vi "ziExample-PollData.vi"(0 "Address":string="DEV", 1 "stop":bool, 5 "Save":bool) -> (17 "theta (deg)":dbl[](array[numeric]), 20 "Selected Device":string, 21 "Demod R (V)":dbl format="%_4p", 22 "Demod Phi (deg)":dbl format="%.3p", 23 "Spectral Density\nVrms/sqrt(Hz)":dbl=1.331104953906021e-08 format="%0.2p", 24 "Savedas":string, 25 "Demod Sample Out":T3 {"Aux In 1 (V)" format="%#_5p"; "Aux In 0 (V)" format="%#_5p"; "X (Vrms)" format="%#_5p"; "Y (Vrms)" format="%#_5p"; "Osc Phase (rad)" format="%#.3g"}, 26 "DIO Out":T2, 27 "AuxIn Out":T1)   [LabVIEW 2009]
doc: "Control a Zurich instrument device via the LabOne Labview API. \nRequirements: Zurich Instruments MFLI, HF2 or UHFLI \nThis example polls data from the instrument.\n\n© Zurich Instruments AG, www.zhinst.com"
uses:
  <instrlib>/Zurich Instruments LabOne/Public/Data/ziTypePollType.ctl
  <instrlib>/Zurich Instruments LabOne/Public/Data/ziTypeDemodSampleEx.ctl
  <instrlib>/Zurich Instruments LabOne/Public/Data/ziTypeAuxInSample.ctl
  <instrlib>/Zurich Instruments LabOne/Public/Configure/ziSetValueDoubleArray.vi
  <instrlib>/Zurich Instruments LabOne/Public/Data/ziGetEventAuxInSample.vi
  <instrlib>/Zurich Instruments LabOne/Public/Data/ziGetEventDemodSample.vi
  <instrlib>/Zurich Instruments LabOne/Public/Data/ziGetEventDIOSample.vi
  <instrlib>/Zurich Instruments LabOne/Zurich Instruments LabOne.lvlib
panel:
  out "data":cluster{dbl[], u32[], dbl[]}
  out "Error Out":errorcluster
  in  "Saveas":path
  in  "Edge":u16(ring)=1 items=["Off", "Rising Edge", "Falling Edge", "Both Edges"]
  in  "DIO Channel":u16(ring) items=["Continous"=0, "DIO 0 / Tigger 3"=1, "DIO 1 / Tigger 4"=4, "DIO 0|1 / Tigger 3|4"=5]
  in  "binSave":bool caption="Binary Save"
  out "Buffer Overflow":bool
  out "Demod sample":dbl[](graph)
  out "ziValueType":T4
  out "DIO":u32[](graph)
  out "AUX Input":dbl[](graph)
  # "ziExample-PollData.vi\nRequirements: HF2, UHFLI or MFLI\nsee block diagram for VI description"
  # "Tested Instruments:\n- MFLI\n- HF2LI\n- UHFLI"
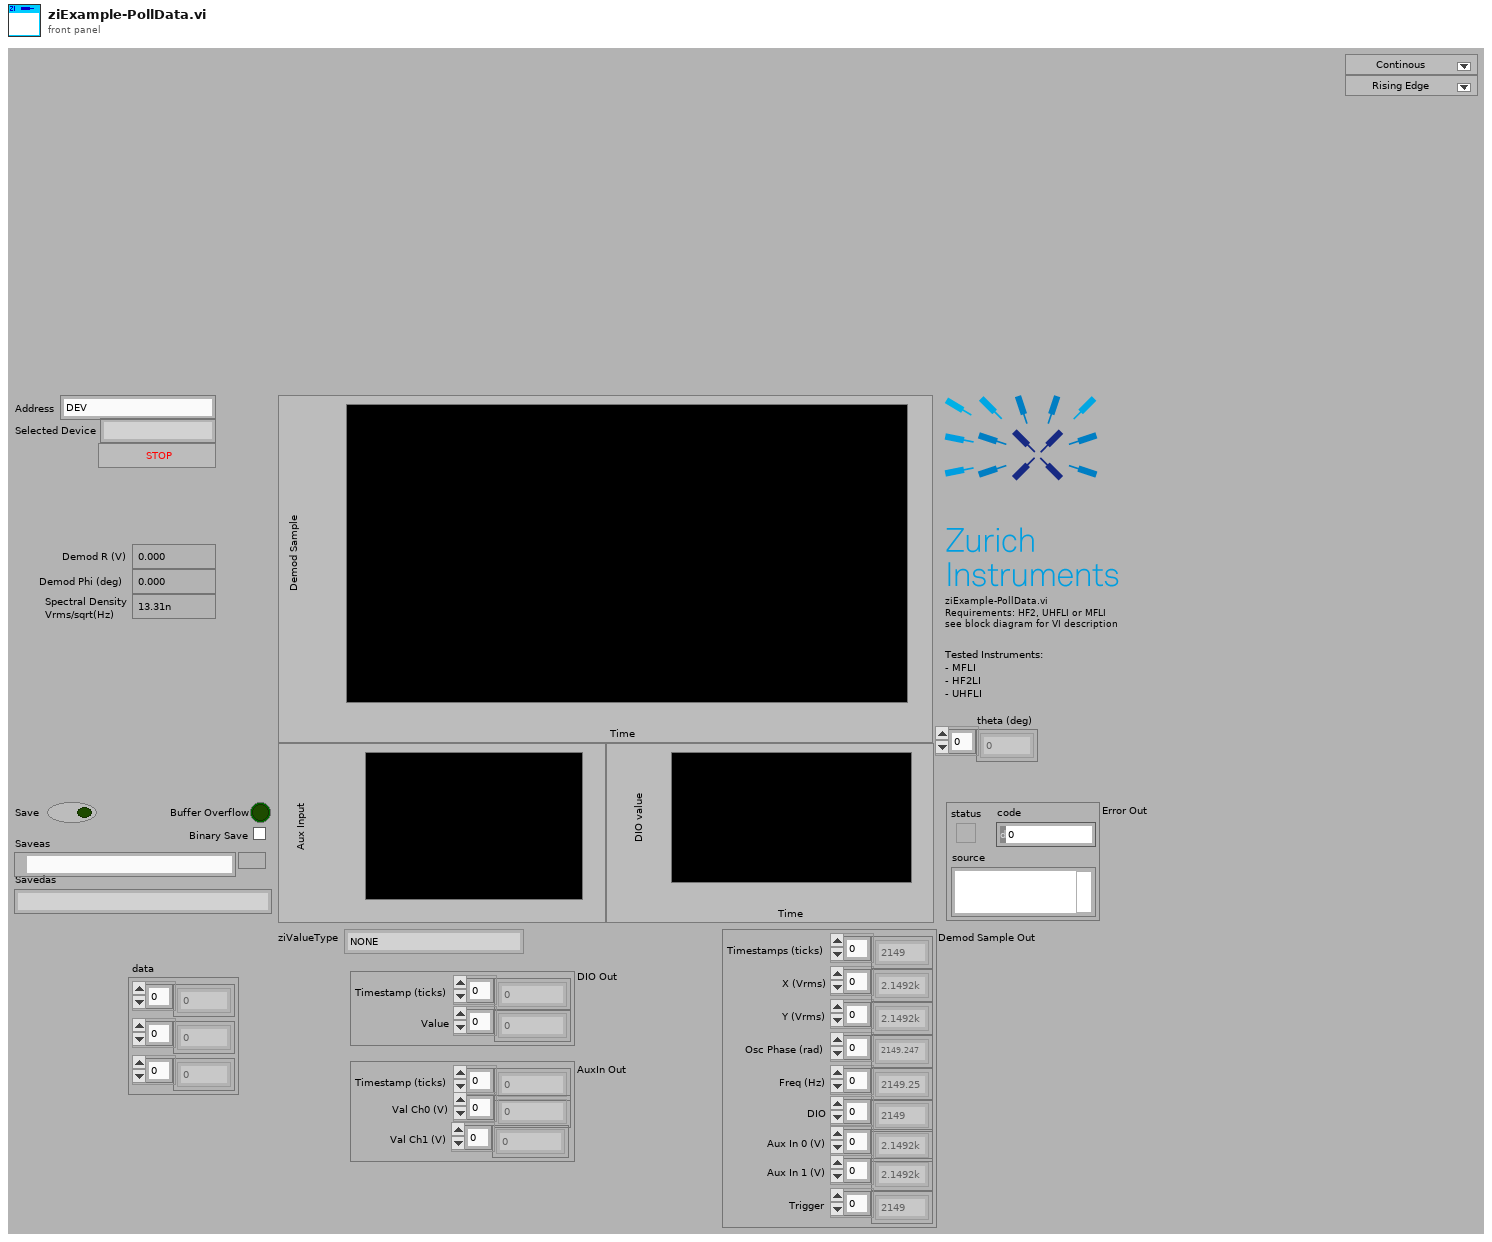
[diagram p1: front panel]
types:
  T1 = typedef "Zurich Instruments LabOne.lvlib/ziTypeAuxInSample.ctl" = cluster{"Timestamp (ticks)":u64[], "Val Ch0 (V)":dbl[], "Val Ch1 (V)":dbl[]}
  T2 = cluster{"Timestamp (ticks)":u64[], "Value":u32[]}
  T3 = typedef "ziTypeDemodSampleEx.ctl" = cluster{"Timestamps (ticks)":u64[], "X (Vrms)":dbl[], "Y (Vrms)":dbl[], "Osc Phase (rad)":dbl[], "Freq (Hz)":dbl[], "DIO":u32[], "Aux In 0 (V)":dbl[], "Aux In 1 (V)":dbl[], "Trigger":u32[]}
  T4 = typedef "Zurich Instruments LabOne.lvlib/ziTypePollType.ctl" = enum16{"NONE", "DOUBLE_DATA", "INTEGER_DATA", "DEMOD_SAMPLE", "SCOPE_WAVE_HF2", "AUXIN_SAMPLE", "DIO_SAMPLE", "BYTE_ARRAY", "PWA_WAVE", "9", "10", "11", "12", "13", "14", "15", "TREE_CHANGE_DEPRI", "17", "ERROR", "19", "20", "21", "22", "23", "24", "25", "26", "27", "28", "29", "30", "31", "DOUBLE_DATA_TS", "INTEGER_DATA_TS", "34", "SCOPE_WAVE", "36", "37", "BYTE_ARRAY_TS", "39", "40", "41", "42", "43", "44", "45", "CNT_DATA", "47", "TREE_CHANGE", "49", "50", "51", "52", "53", "54", "55", "56", "57", "58", "59", "60", "61", "62", "63", "SWEEPER_DATA", "SPECTRUM_DATA", "ADVISOR_DATA", "67", "IMP_DATA"}
  T5 = typedef "Zurich Instruments LabOne.lvlib/ziTypeHandle.ctl" = cluster{"handleValid":bool, "Conn":u64, "Path Prefix":string, "Handle":u64, "Connected":bool, "Clockbase(s)":dbl}
  T6 = enum16{"open", "replace", "create", "open or create", "replace or create", "replace or create with confirmation"}
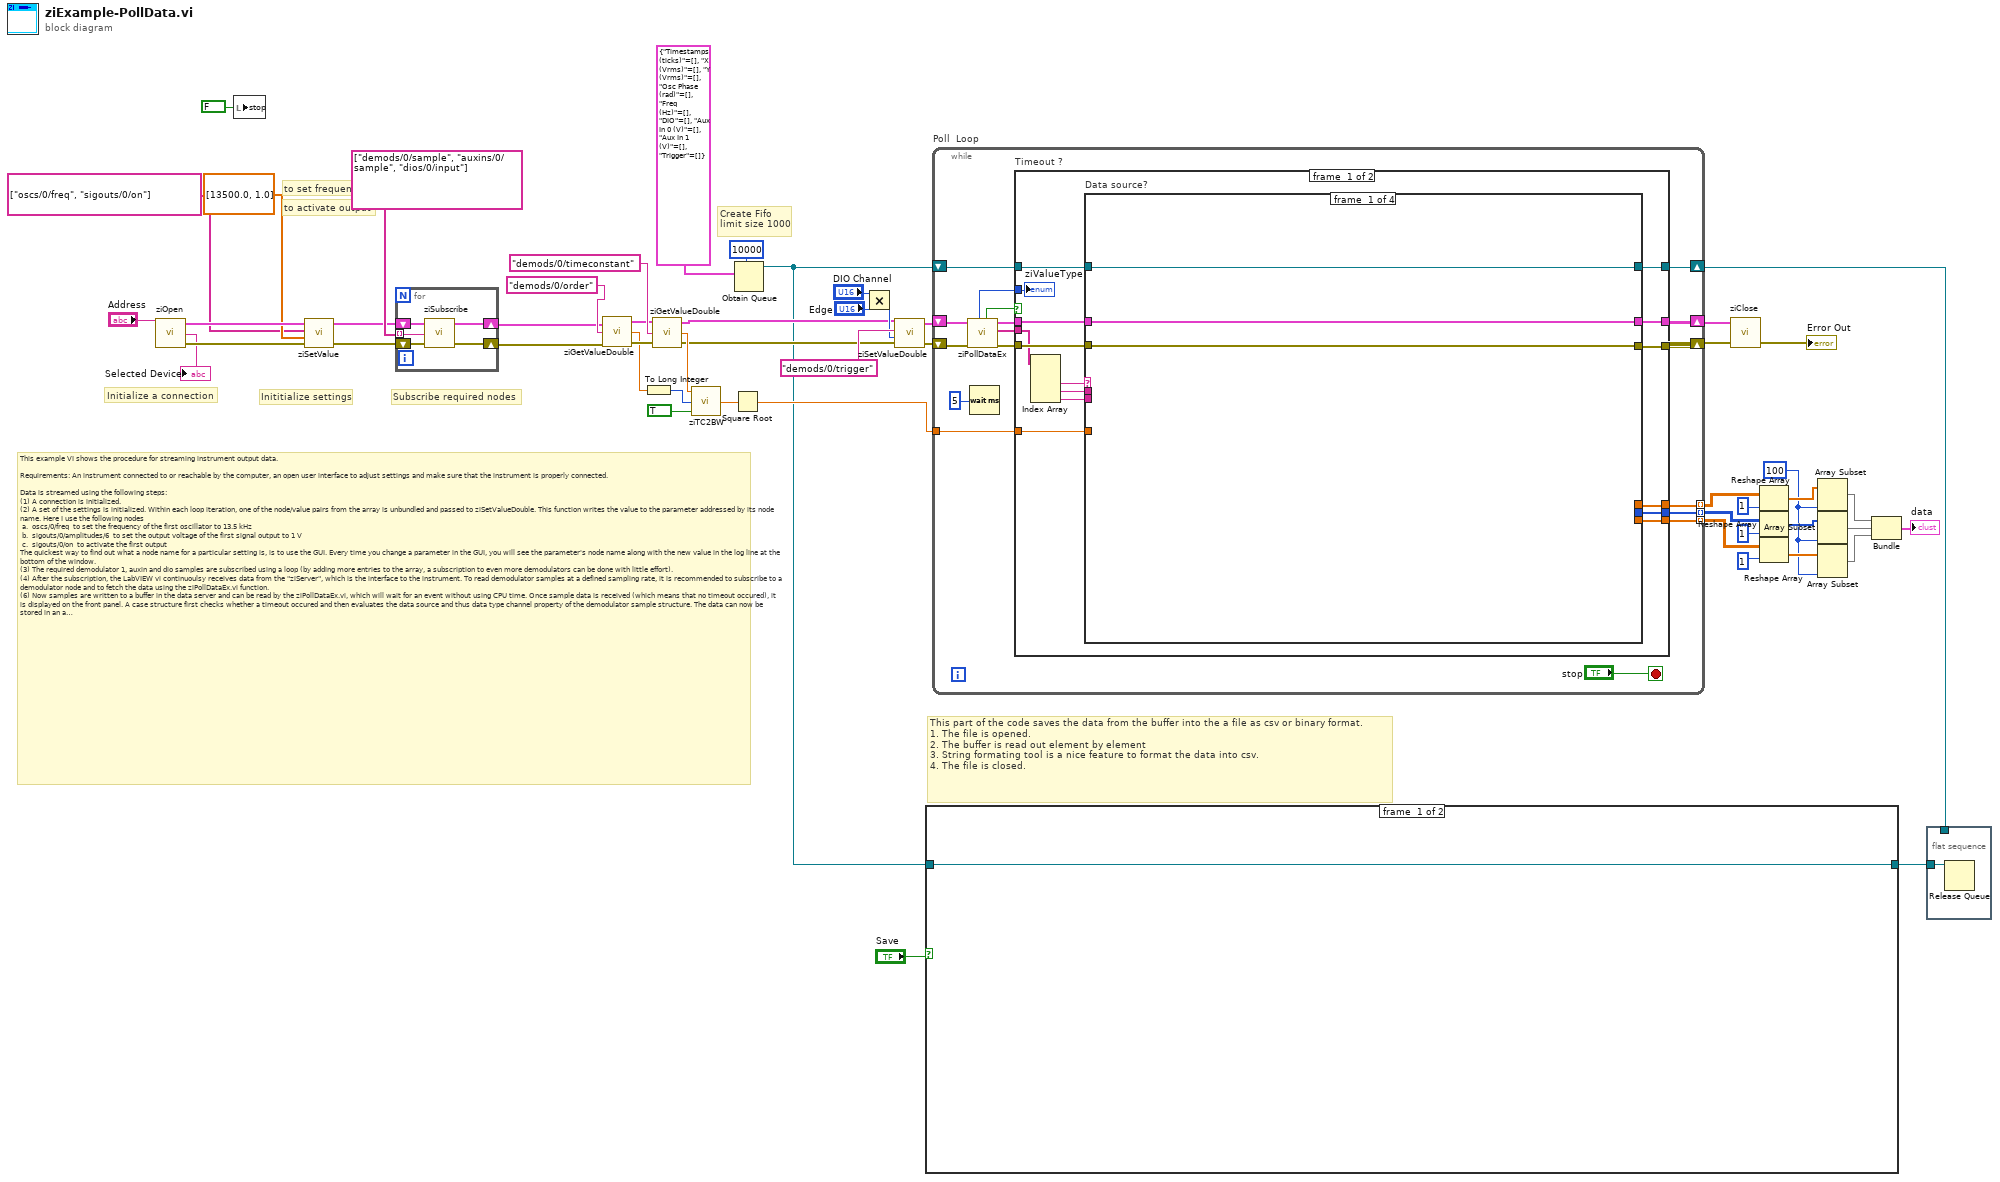
[diagram p0: block diagram]
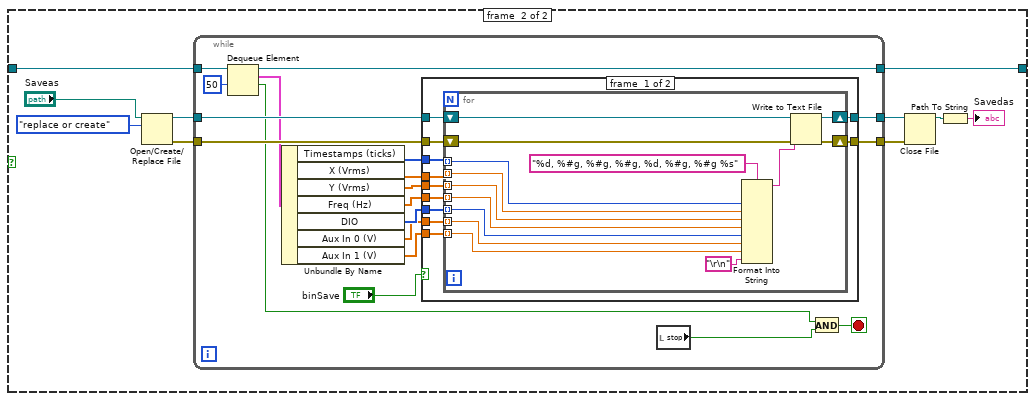
[diagram p2: hidden frame]
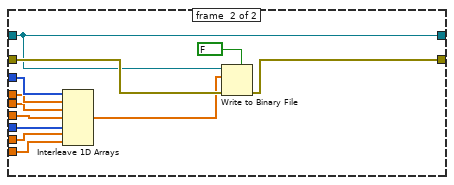
[diagram p3: hidden frame]
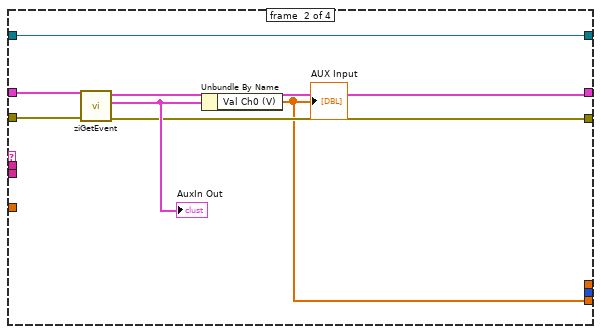
[diagram p4: hidden frame]
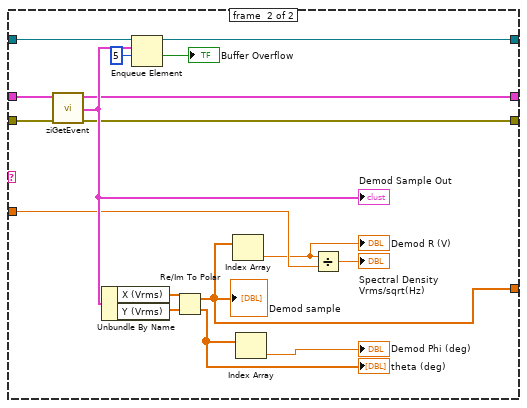
[diagram p7: hidden frame]
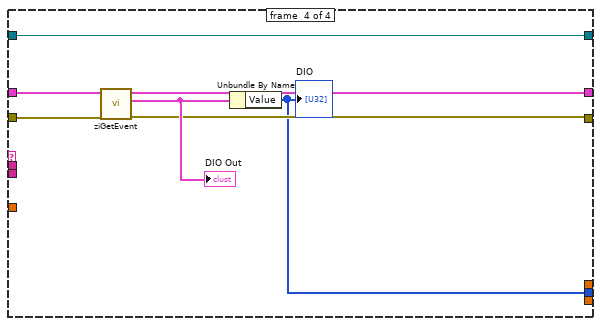
[diagram p8: hidden frame]
diagram:
  w2 = 100 ("dimension size")
  # "This part of the code saves the data from the buffer into the a file as csv or binary format. \n1. The file is opened.\n2. The buffer is read out element by element\n3. String formating tool is a nice feature to format the data into csv.\n4. The file is closed."
  # "Create Fifo\nlimit size 1000"
  # "to activate output"
  # "to set frequency"
  # "Inititialize settings"
  # "Initialize a connection"
  # "Subscribe required nodes"
  # "This example VI shows the procedure for streaming instrument output data.\n\nRequirements: An instrument connected to or reachable by the computer, an open user interface to adjust settings and make sure that the instrument is properly connected. \n\nData is streamed using the following steps:\n(1) A connection is initialized.\n(2) A set of the settings is initialized. Within each loop iteration, one of the node/value pairs from the array is unbundled and passed to ziSetValueDouble. This function writes the value to the parameter addressed by its node name. Here I use the following nodes\n a. \toscs/0/freq \tto set the frequency of the first oscillator to 13.5 kHz\n b. \tsigouts/0/amplitudes/6 \tto set the output voltage of the first signal output to 1 V\n c. \tsigouts/0/on \tto activate the first output\nThe quickest way to find out what a node name for a particular setting is, is to use the GUI. Every time you change a parameter in the GUI, you will see the parameter's node name along with the new value in the log line at the bottom of the window. \n(3) The required demodulator 1, auxin and dio samples are subscribed using a loop (by adding more entries to the array, a subscription to even more demodulators can be done with little effort).\n(4) After the subscription, the LabVIEW vi continuoulsy receives data from the \"ziServer\", which is the interface to the instrument. To read demodulator samples at a defined sampling rate, it is recommended to subscribe to a demodulator node and to fetch the data using the ziPollDataEx.vi function. \n(6) Now samples are written to a buffer in the data server and can be read by the ziPollDataEx.vi, which will wait for an event without using CPU time. Once sample data is received (which means that no timeout occured), it is displayed on the front panel. A case structure first checks whether a timeout occured and then evaluates the data source and thus data type channel property of the demodulator sample structure. The data can now be stored in an array or a queue or be shown in a waveform chart. \n(7) Finally, the connection is closed. \n \n© Zurich Instruments AG, 2016, www.zhinst.com"
  n1 = call <instrlib>:"ziOpen.vi"("Address"="Address") -> ("Error Out"=w49:errorcluster, "Selected Device"=→"Selected Device":string, "HandleOut"=w48:T5)  [unwired: 1 in, 2 out]
  n2 = local write "stop"(FALSE ("stop")) -> ()
  n3 = call-poly <instrlib>:"ziSetValue.vi"("Error In"=w49, "Values"=dbl[] [13500.0, 1.0], "Paths"=string[] ["oscs/0/freq", "sigouts/0/on"], "Handle In"=w48) -> ("Error Out"=w50:errorcluster, "Handle Out"=w51:T5)  [unwired: 1 in]
  n4 = for {
    shift-right: [w58] -> w32
    shift-left: w51 -> [w56]
    shift-right: [w57] -> w31
    shift-left: w50 -> [w55]
    tunnel: string[] ["demods/0/sample", "auxins/0/sample", "dios/0/input"] -> [w54] mode=indexing
    n5 = call <instrlib>:"ziSubscribe.vi"("error in"=w55, "Path ()"=w54, "Handle In"=w56) -> ("error out"=w57:errorcluster, "Handle Out"=w58:T5)  [unwired: 1 in]
  }
  n6 = call <instrlib>:"ziGetValueDouble.vi"("error in"=w31, "Path"="demods/0/order", "Handle in"=w32) -> ("error out"=w38:errorcluster, "Value"=w37:dbl, "Handle out"=w39:T5)
  n7 = To Long Integer(number=w37) -> (32bit integer=w36:i32)
  n8 = call <instrlib>:"ziGetValueDouble.vi"("error in"=w38, "Path"="demods/0/timeconstant", "Handle in"=w39) -> ("error out"=w19:errorcluster, "Value"=w35:dbl, "Handle out"=w20:T5)
  n9 = call <instrlib>:"ziTC2BW.vi"("Eq BW (F)"=TRUE ("Eq BW"), "Order (1)"=w36, "TC (s)"=w35) -> ("BW (Hz)"=w34:dbl)
  n10 = Square Root(x=w34) -> (sqrt(x)=w30:dbl)
  n11 = Obtain Queue(max queue size (-1, unlimited)=10000, element data type=T3 {"Timestamps (ticks)"=[], "X (Vrms)"=[], "Y (Vrms)"=[], "Osc Phase (rad)"=[], "Freq (Hz)"=[], "DIO"=[], "Aux In 0 (V)"=[], "Aux In 1 (V)"=[], "Trigger"=[]} ("Demod Sample Out")) -> (queue out=w18:refnum<queue>)  [unwired: 3 in, 2 out]
  n12 = Multiply(x="DIO Channel", y="Edge") -> (x*y=w25:u16)
  n13 = call <instrlib>:"ziSetValueDouble.vi"("Error In"=w19, "Value"=w25, "Path"="demods/0/trigger", "Handle In"=w20) -> ("Error Out"=w22:errorcluster, "Handle Out"=w21:T5)  [unwired: 1 in]
  n14 = case shown="True" "Save" {
    tunnel: w18 -> [w59 w69]
    tunnel: [w59 w64] -> w28
    frame #0 {
    }
    frame #1 {
      n15 = Open/Create/Replace File(file path (use dialog)="Saveas", operation (0:open)=T6."replace or create") -> (refnum out=w67:refnum<file>, error out=w68:errorcluster)  [unwired: 4 in, 1 out]
      n16 = while {
        tunnel: w68 -> [w81]
        tunnel: w67 -> [w80]
        tunnel: [w79] -> w66
        tunnel: [w78] -> w65
        tunnel: [w73] -> w64
        tunnel: w69 -> [w75]
        stop <- w71 stop-if-true
        n17 = Dequeue Element(queue=w75, timeout in ms (-1)=50) -> (queue out=w73:refnum<queue>, element=w76:T3, timed out?=w74:bool)  [unwired: 1 in, 1 out]
        n18 = Unbundle By Name(w76) -> ("Timestamps (ticks)"=w88:u64[], "X (Vrms)"=w85:dbl[], "Y (Vrms)"=w87:dbl[], "Freq (Hz)"=w86:dbl[], "DIO"=w84:u32[], "Aux In 0 (V)"=w83:dbl[], "Aux In 1 (V)"=w82:dbl[])
        n19 = case shown="False" "binSave" {
          tunnel: w88 -> [w99 w121]
          tunnel: w87 -> [w98 w119]
          tunnel: w86 -> [w97 w118]
          tunnel: w85 -> [w96 w120]
          tunnel: w84 -> [w95 w117]
          tunnel: w83 -> [w94 w116]
          tunnel: w82 -> [w93 w115]
          tunnel: w81 -> [w92 w124]
          tunnel: w80 -> [w91 w122]
          tunnel: [w90 w123] -> w79
          tunnel: [w89 w122] -> w78
          frame #0 {
            n20 = for {
              tunnel: w99 -> [w107] mode=indexing
              tunnel: w98 -> [w105] mode=indexing
              tunnel: w96 -> [w106] mode=indexing
              shift-right: [w112] -> w89
              shift-left: w91 -> [w113]
              tunnel: w97 -> [w104] mode=indexing
              shift-right: [w111] -> w90
              shift-left: w92 -> [w110]
              tunnel: w95 -> [w102] mode=indexing
              tunnel: w94 -> [w101] mode=indexing
              tunnel: w93 -> [w103] mode=indexing
              n21 = Format Into String(format string="%d, %#g, %#g, %#g, %d, %#g, %#g %s", w107, w106, w105, w104, w102, w101, w103, "\r\n") -> (resulting string=w100:string)  [unwired: 2 in, 1 out]
              n22 = Write to Text File(file (use dialog)=w113, text=w100, error in=w110) -> (refnum out=w112:refnum<file>, error out=w111:errorcluster)  [unwired: 2 out]
            }
          }
          frame #1 {
            n23 = Interleave 1D Arrays(w121, w120, w119, w118, w117, w116, w115) -> (w114:dbl[])
            n24 = Write to Binary File(file (use dialog)=w122, data=w114, error in=w124, 5:FALSE ("prepend array or string size? (T)")) -> (error out=w123:errorcluster)  [unwired: 4 out]
          }
        }
        n25 = local read "stop"() -> (w72:bool)
        n26 = And(x=w74, y=w72) -> (x .and. y?=w71:bool)
      }
      n27 = Close File(refnum=w65, error in=w66) -> (path=w61:path)  [unwired: 1 out]
      n28 = Path To String(path=w61) -> (string=→"Savedas":string)
    }
  }
  n29 = while "Poll  Loop" {
    shift-right: [w142] -> w53
    shift-left: w21 -> [w130]
    shift-right: [w138] -> w29
    shift-left: w22 -> [w129]
    shift-right: [w134] -> w17
    shift-left: w18 -> [w135]
    tunnel: w30 -> [w133]
    tunnel: [w128] -> w7 mode=indexing
    tunnel: [w127] -> w8 mode=indexing
    tunnel: [w126] -> w9 mode=indexing
    stop <- "stop" stop-if-true
    n30 = call <instrlib>:"ziPollDataEx.vi"("error in"=w129, "Handle In"=w130) -> ("error out"=w139:errorcluster, "PathArray"=w136:string[], "Handle Out"=w141:T5, "Timed Out"=w140:bool, "ziValueType"=w137:T4)  [unwired: 2 in, 3 out]
    n31 = Wait (ms)(milliseconds to wait=u32 5) -> ()  [unwired: 1 out]
    n32 = case "Timeout ?" shown="True" w140 {
      tunnel: w141 -> [w157 w219]
      tunnel: [w156 w219] -> w142
      tunnel: w139 -> [w155 w218]
      tunnel: [w154 w218] -> w138
      tunnel: w137 -> [w153 _]
      tunnel: w136 -> [w152 _]
      tunnel: [w148 w217] -> w134
      tunnel: w135 -> [w147 w217]
      tunnel: w133 -> [w146 _]
      tunnel: [w145 _] -> w128
      tunnel: [w144 _] -> w127
      tunnel: [w143 _] -> w126
      frame #0 {
        n33 = Index Array(array=w152) -> (element #2=w149:string, element #3=w150:string, element #4=w151:string)  [unwired: 4 in, 1 out]
        n34 = case "Data source?" shown="\"DEMODS\"" w149 {
          tunnel: w157 -> [w160 w167 w177 w216]
          tunnel: [w160 w165 w176 w215] -> w156
          tunnel: w155 -> [w159 w164 w175 w213]
          tunnel: [w159 w163 w174 w212] -> w154
          tunnel: w150 -> [_ _ w173 _]
          tunnel: w151 -> [_ _ w172 _]
          tunnel: [w158 w162 w171 w211] -> w148
          tunnel: w147 -> [w158 w162 w170 w211]
          tunnel: w146 -> [_ _ w169 _]
          tunnel: [_ _ w168 _] -> w145
          tunnel: [_ _ _ w210] -> w144
          tunnel: [_ w161 _ _] -> w143
          frame #0 {
          }
          frame #1 {
            n35 = call-poly <instrlib>:"ziGetEvent.vi"("Error In"=w164, "Handle In"=w167) -> ("Error Out"=w163:errorcluster, "AuxIn Out"=w166:T1, "Handle Out"=w165:T5)  [unwired: 7 in]
            "AuxIn Out" <- w166
            n36 = Unbundle By Name(w166) -> ("Val Ch0 (V)"=w161:dbl[])
            "AUX Input" <- w161
          }
          frame #2 {
            n37 = case shown="\"0\"" w173 {
              tunnel: w177 -> [w180 w189]
              tunnel: [w180 w188] -> w176
              tunnel: w175 -> [w179 w187]
              tunnel: [w179 w186] -> w174
              tunnel: w172 -> [_ w185]
              tunnel: [w178 w184] -> w171
              tunnel: w170 -> [w178 w183]
              tunnel: w169 -> [_ w182]
              tunnel: [_ w181] -> w168
              frame #0 {
              }
              frame #1 {
                n38 = case shown="\"SAMPLE\"" w185 {
                  tunnel: w189 -> [w192 w207]
                  tunnel: [w192 w201] -> w188
                  tunnel: w187 -> [w191 w206]
                  tunnel: [w191 w200] -> w186
                  tunnel: [w190 w198] -> w184
                  tunnel: w183 -> [w190 w205]
                  tunnel: w182 -> [_ w202]
                  tunnel: [_ w196] -> w181
                  frame #0 {
                  }
                  frame #1 {
                    n39 = call-poly <instrlib>:"ziGetEvent.vi"("Error In"=w206, "Handle In"=w207) -> ("Error Out"=w200:errorcluster, "Demod Sample Out"=w204:T3, "Handle Out"=w201:T5)  [unwired: 7 in]
                    "Demod Sample Out" <- w204
                    n40 = Unbundle By Name(w204) -> ("X (Vrms)"=w209:dbl[], "Y (Vrms)"=w208:dbl[])
                    n41 = Enqueue Element(queue=w205, element=w204, timeout in ms (-1)=5) -> (queue out=w198:refnum<queue>, timed out?=→"Buffer Overflow":bool)  [unwired: 1 in, 1 out]
                    n42 = Re/Im To Polar(2:w208, 3:w209) -> (0:w195:dbl[], 1:w196:dbl[])
                    "Demod sample" <- w196
                    "theta (deg)" <- w195
                    n43 = Index Array(array=w196) -> (element=w193:dbl)  [unwired: 1 in]
                    "Demod R (V)" <- w193
                    n44 = Index Array(array=w195) -> (element=→"Demod Phi (deg)":dbl)  [unwired: 1 in]
                    n45 = Divide(x=w193, y=w202) -> (x/y=→"Spectral Density\nVrms/sqrt(Hz)":dbl)
                  }
                }
              }
            }
          }
          frame #3 {
            n46 = call-poly <instrlib>:"ziGetEvent.vi"("Error In"=w213, "Handle In"=w216) -> ("Error Out"=w212:errorcluster, "DIO Out"=w214:T2, "Handle Out"=w215:T5)  [unwired: 7 in]
            "DIO Out" <- w214
            n47 = Unbundle By Name(w214) -> ("Value"=w210:u32[])
            "DIO" <- w210
          }
        }
        "ziValueType" <- w153
      }
      frame #1 {
        # "Timeout, no action."
      }
    }
  }
  n48 = call <instrlib>:"ziClose.vi"("Error In"=w29, "Handle In"=w53) -> ("Error Out"=→"Error Out":errorcluster)  [unwired: 3 out]
  n49 = Reshape Array(w7, 1 ("dimension size")) -> (w6:dbl[])
  n50 = Reshape Array(w8, 1 ("dimension size")) -> (w5:u32[])
  n51 = Reshape Array(w9, 1 ("dimension size")) -> (w4:dbl[])
  n52 = Array Subset(array=w6, length=w2) -> (w14:dbl[])  [unwired: 1 in]
  n53 = Array Subset(array=w5, length=w2) -> (w13:u32[])  [unwired: 1 in]
  n54 = Array Subset(array=w4, length=w2) -> (w3:dbl[])  [unwired: 1 in]
  n55 = Bundle(w14, w13, w3) -> (→"data":cluster{dbl[], u32[], dbl[]})  [unwired: 1 in]
  n56 = flat-sequence {
    tunnel: w28 -> [w220]
    tunnel: w17 -> [_]
    frame #0 {
      n57 = Release Queue(queue=w220) -> ()  [unwired: 2 in, 3 out]
    }
  }
